vi "GET_1BIT.vi"(6 "wait for reply (T)":bool=TRUE, 8 "error in (no error)":errorcluster, 10 "GET 1BIT":u8, 11 "Module ID":i32=-1) -> (0 "error out":errorcluster, 1 "timed out?":bool, 2 "Reply Payload":T1)   [LabVIEW 2019, in "Multiple_uC.lvlib"]
doc: "Obtain the value of 1 specific bit of the input of the microcontroller\n_____\nCreated using Delacor QMH Event Scripter 5.0.0.112."
uses:
  Multiple_uC.lvlib
  GET_1BIT (Reply Payload)--cluster.ctl
  GET_1BIT Argument--cluster.ctl
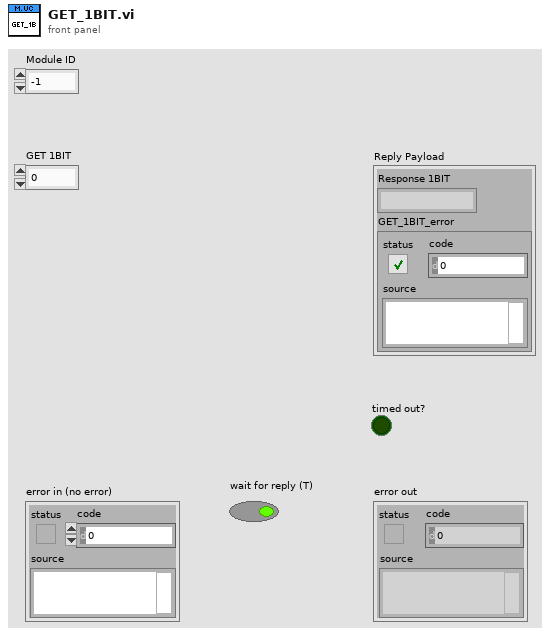
[diagram p1: front panel]
types:
  T1 = typedef "Multiple_uC.lvlib/GET_1BIT (Reply Payload)--cluster.ctl" = cluster{"Response 1BIT":string, "GET_1BIT_error":errorcluster}
  T2 = typedef "Multiple_uC.lvlib/GET_1BIT Argument--cluster.ctl" = cluster{"Module ID":i32, "GET 1BIT":u8, "Wait Notifier":refnum<notifier>, "wait for reply":bool}
  T3 = typedef "Multiple_uC.lvlib/Request Events--cluster.ctl" = cluster{"Stop Module":refnum<user-event>, "Show Panel":refnum<user-event>, "Hide Panel":refnum<user-event>, "Show Diagram":refnum<user-event>, "Get Module Execution Status":refnum<user-event>, "ADC´s View":refnum<user-event>, "Write_1BIT":refnum<user-event>, "Set 8 bits":refnum<user-event>, "GET_1BIT":refnum<user-event>, "GET_8BITS":refnum<user-event>}
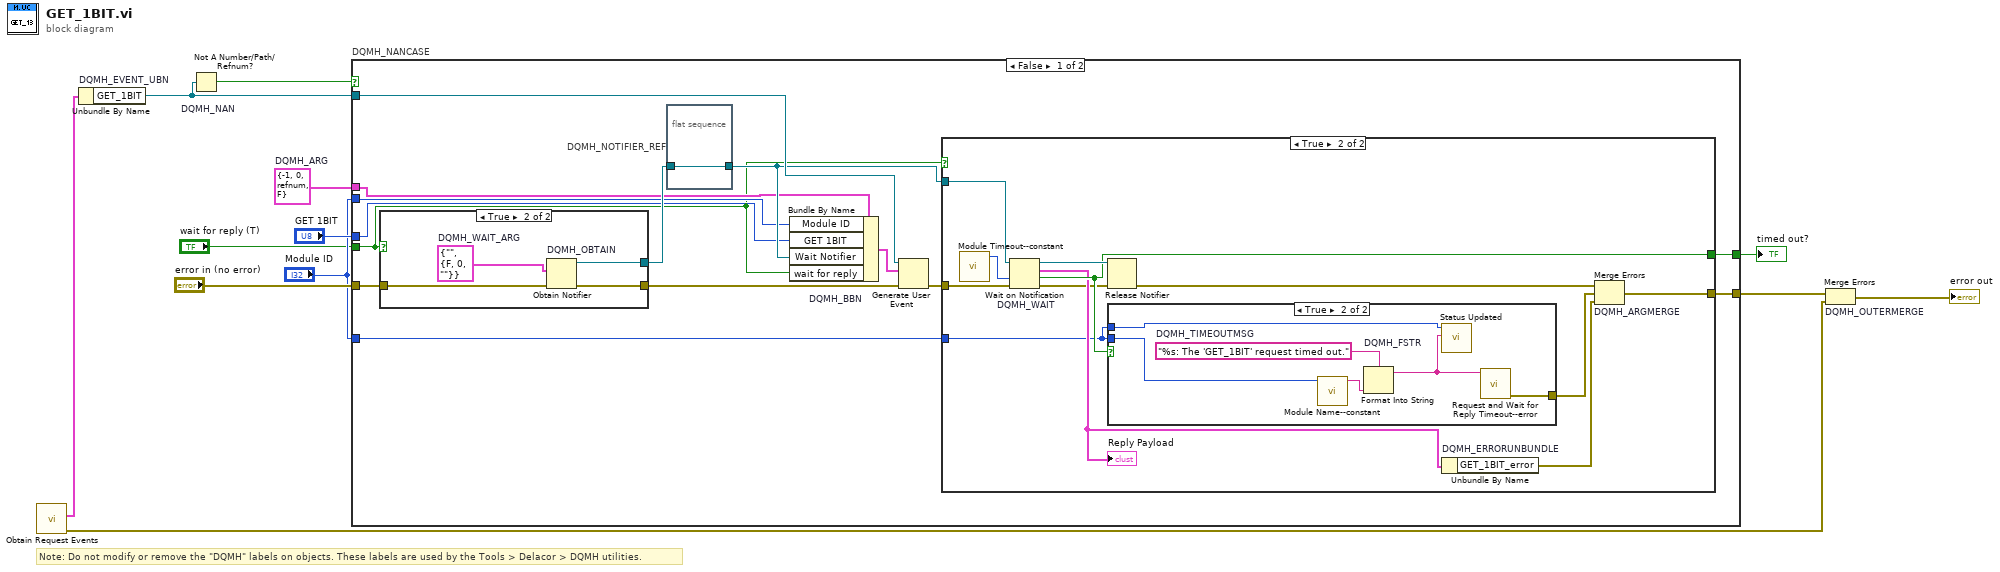
[diagram p0: block diagram]
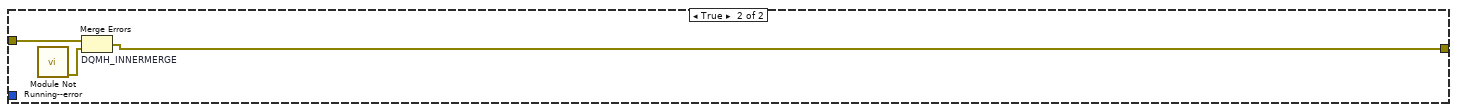
[diagram p5: hidden frame]
diagram:
  w6 = T2 {"Module ID"=-1, "GET 1BIT"=0, "Wait Notifier"=refnum, "wait for reply"=FALSE}  # DQMH_ARG
  # "Note: Do not modify or remove the \"DQMH\" labels on objects. These labels are used by the Tools > Delacor > DQMH utilities."
  n1 = call "Obtain Request Events.vi"() -> ("error out"=w2:errorcluster, "Multiple_uC Request Events"=w1:T3)  [unwired: 10 in]
  n2 = Unbundle By Name "DQMH_EVENT_UBN"(w1) -> ("GET_1BIT"=w10:refnum<user-event>)
  n3 = Not A Number/Path/Refnum? "DQMH_NAN"(number/path/refnum=w10) -> (NaN/Path/Refnum?=w9:bool)
  n4 = case "DQMH_NANCASE" shown="False" w9 {
    tunnel: "error in (no error)" -> [w26 w54]
    tunnel: w10 -> [w24 _]
    tunnel: [w21 w53] -> w7
    tunnel: [w22 _] -> w8
    tunnel: w6 -> [w17 _]
    tunnel: "Module ID" -> [w16 _]
    tunnel: "GET 1BIT" -> [w15 _]
    tunnel: "Module ID" -> [w14 _]
    tunnel: "wait for reply (T)" -> [w13 _]
    frame False {
      n5 = case shown="True" w13 {
        tunnel: w26 -> [w47 w51]
        tunnel: [w47 w50] -> w23
        tunnel: [_ w48] -> w19
        frame False {
        }
        frame True {
          w49 = T1 {"Response 1BIT"="", "GET_1BIT_error"={"status"=FALSE, "code"=0, "source"=""}}  # DQMH_WAIT_ARG
          n6 = Obtain Notifier "DQMH_OBTAIN"(notification data type=w49, error in (no error)=w51) -> (notifier out=w48:refnum<notifier>, error out=w50:errorcluster)  [unwired: 2 in, 1 out]
        }
      }
      n7 = flat-sequence "DQMH_NOTIFIER_REF" {
        tunnel: w19 -> [w27]
        tunnel: [w27] -> w18
        frame #0 {
        }
      }
      n8 = Bundle By Name "DQMH_BBN"(cluster=w17, "Module ID"=w16, "GET 1BIT"=w15, "Wait Notifier"=w18, "wait for reply"=w13) -> (w20:T2)
      n9 = Generate User Event(user event=w24, event data cluster=w20, error in=w23) -> (error out=w25:errorcluster)  [unwired: 1 in, 1 out]
      n10 = case shown="True" w13 {
        tunnel: w25 -> [w28 w40]
        tunnel: w18 -> [_ w39]
        tunnel: [_ w37] -> w22
        tunnel: [w28 w36] -> w21
        tunnel: w14 -> [_ w29]
        frame False {
        }
        frame True {
          n11 = call "Module Timeout--constant.vi"() -> ("Module Timeout"=w30:i32)  [unwired: 11 in]
          n12 = Wait on Notification "DQMH_WAIT"(notifier=w39, timeout in ms (-1)=w30, error in (no error)=w40) -> (notifier out=w38:refnum<notifier>, notification=w35:T1, timed out?=w37:bool, error out=w34:errorcluster)  [unwired: 1 in]
          "Reply Payload" <- w35
          n13 = Release Notifier(notifier=w38, error in (no error)=w34) -> (error out=w33:errorcluster)  [unwired: 1 in, 2 out]
          n14 = case shown="True" w37 {
            tunnel: [_ w44] -> w31
            tunnel: w29 -> [_ w42]
            tunnel: w29 -> [_ w41]
            frame False {
            }
            frame True {
              w46 = "%s: The 'GET_1BIT' request timed out."  # DQMH_TIMEOUTMSG
              n15 = call "Module Name--constant.vi"("Module ID"=w41) -> ("Module Name"=w43:string)  [unwired: 10 in]
              n16 = Format Into String "DQMH_FSTR"(format string=w46, w43) -> (resulting string=w45:string)  [unwired: 2 in, 1 out]
              n17 = call "Status Updated.vi"("Status"=w45, "Module ID"=w42) -> ()  [unwired: 9 in, 1 out]
              n18 = call "Request and Wait for Reply Timeout--error.vi"("Error Message"=w45) -> ("error out"=w44:errorcluster)  [unwired: 10 in]
            }
          }
          n19 = Unbundle By Name "DQMH_ERRORUNBUNDLE"(w35) -> ("GET_1BIT_error"=w32:errorcluster)
          n20 = Merge Errors "DQMH_ARGMERGE"(w33, w31, w32) -> (w36:errorcluster)
        }
      }
    }
    frame True {
      n21 = call "Module Not Running--error.vi"() -> ("error out"=w52:errorcluster)  [unwired: 11 in]
      n22 = Merge Errors "DQMH_INNERMERGE"(w54, w52) -> (w53:errorcluster)
    }
  }
  "timed out?" <- w8
  n23 = Merge Errors "DQMH_OUTERMERGE"(w7, w2) -> (→"error out":errorcluster)
